vi "Auto.vi"(8 "error in (no error)":errorcluster, 11 "PID in":refnum<class "PID.lvclass">) -> (0 "error out":errorcluster, 3 "PID out":refnum<class "PID.lvclass">)   [LabVIEW 2025, in "PID.lvlib" / "PID.lvclass"]
uses:
  PID.lvclass
  PID.lvclass/PID.ctl
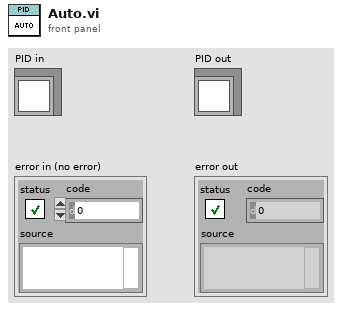
[diagram p1: front panel]
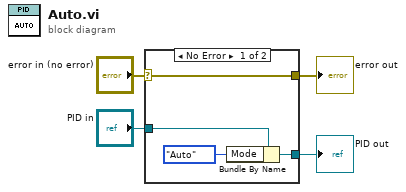
[diagram p0: block diagram]
diagram:
  n1 = case shown="No Error" "error in (no error)" {
    selector: "error in (no error)" -> [w8 w10]
    tunnel: [w8 w10] -> w3
    tunnel: [w6 w9] -> w1
    tunnel: "PID in" -> [w7 w9]
    frame No Error {
      n2 = Bundle By Name(cluster=w7, "Mode"=enum16{"Manual", "Auto"}."Auto") -> (w6:refnum<class "PID.lvclass">)
    }
    frame Error {
    }
  }
  "error out" <- w3
  "PID out" <- w1
